vi "Execute.vi"(8 "error in (no error)":errorcluster, 10 "Shifted Error in":refnum<class "Error.lvclass">, 11 "ERROR_Prompt in":refnum<class "ERROR_Prompt.lvclass">) -> (0 "error out":errorcluster, 1 "STOP?":bool, 2 "Shifted Error out":refnum<class "Error.lvclass">, 3 "ERROR_Prompt out":refnum<class "ERROR_Prompt.lvclass">)   [LabVIEW 2019, in "TSC Error.lvlib" / "ERROR_Prompt.lvclass"]
doc: "The Error Prompt function will send a message using the queue reference to the application for the error that happened in the software.\n\nInputs:\n-ERROR_Prompt in [obj] - the dynamic dispatch input class\n-Shifted Error in [obj] - the shifted error class with shared information\n-error in\n\nOutputs:\n-ERROR_Prompt out [obj] - the dynamic dispatch output class\n-Shifted Error in [obj] - the shifted error class with shared information\n-STOP? [Boolean] - the output Boolean used to stop the Error Loop\n-error out\n\n<b>Code Developed By:</b>\nDaniel Coons\nTechnology Service Corporation\n1983 S Liberty Drive\nBloomington, IN 47403\nPhone: 812 558-7100\nwww.tsc.com\\atcs"
uses:
  ERROR_Prompt.lvclass
  C:/Development/Open Source/tsc-error-library/_Messages/Error/Error.lvclass
  Error/Error.lvclass
  <vilib>/Utility/error.llb/DialogType.ctl
  Error/Error.lvclass/Error.ctl
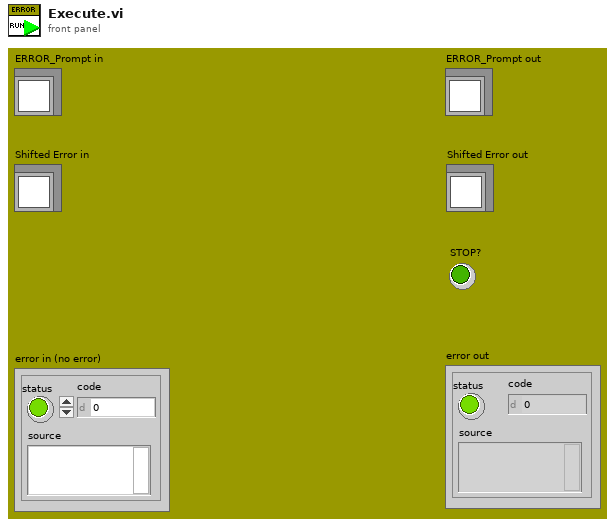
[diagram p1: front panel]
types:
  T1 = typedef "DialogType.ctl" = u16
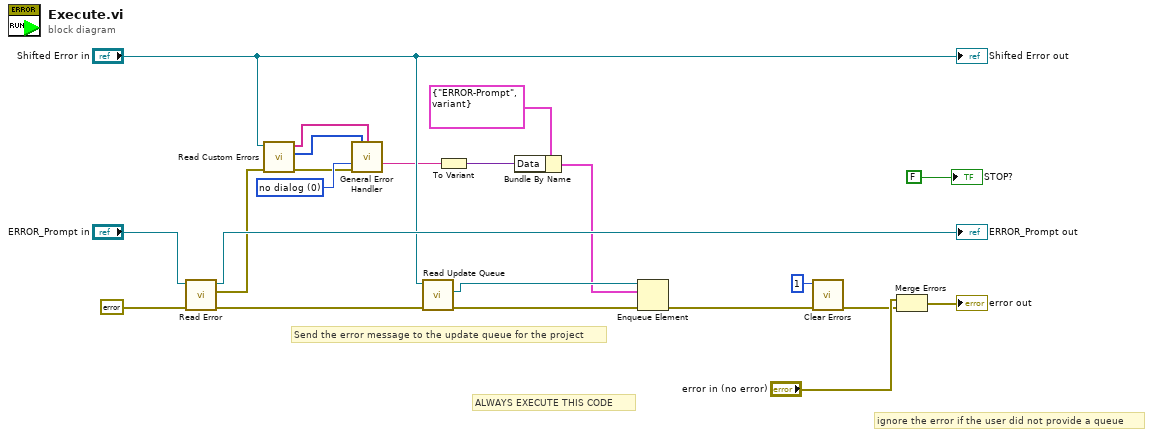
[diagram p0: block diagram]
diagram:
  w20 = T1 0 items=["no dialog", "OK message", "continue or stop message", "OK message + warnings", "continue/stop + warnings"] ("type of dialog (OK msg:1)")
  # "ignore the error if the user did not provide a queue"
  # "Send the error message to the update queue for the project"
  # "ALWAYS EXECUTE THIS CODE"
  n1 = call "Read Error.vi"("error in"=errorcluster {"status"=FALSE, "code"=0, "source"=""} ("error in (no error)"), "Error in"="ERROR_Prompt in") -> ("error out"=w9:errorcluster, "Error"=w19:errorcluster, "Error out"=→"ERROR_Prompt out":refnum<class "ERROR_Prompt.lvclass">)  [unwired: 7 in]
  n2 = call "Read Custom Errors.vi"("Error In"=w19, "Error.lvclass"="Shifted Error in") -> ("Error Out"=w18:errorcluster, "Error Codes"=w16:i32[], "Error Messages"=w17:string[])  [unwired: 7 in]
  n3 = call <vilib>:"General Error Handler.vi"("[user-defined codes]"=w16, "[user-defined descriptions]"=w17, "type of dialog (OK msg:1)"=w20, "error in (no error)"=w18) -> ("message"=w5:string)  [unwired: 7 in, 4 out]
  n4 = call "Read Update Queue.vi"("error in (no error)"=w9, "Error in"="Shifted Error in") -> ("error out"=w10:errorcluster, "Update Queue"=w7:refnum<queue>)  [unwired: 7 in, 1 out]
  n5 = To Variant(anything=w5) -> (Variant=w4:variant)
  n6 = Bundle By Name(cluster=cluster{"Message":string, "Data":variant} {"Message"="ERROR-Prompt", "Data"=variant} ("element"), "Data"=w4) -> (w3:cluster{"Message":string, "Data":variant})
  n7 = Enqueue Element(queue=w7, element=w3, error in (no error)=w10) -> (error out=w8:errorcluster)  [unwired: 1 in, 2 out]
  n8 = call <vilib>:"Clear Errors.vi"("error in (no error)"=w8, "specific error code to clear (0: all)"=1 ("Error Code")) -> ("error out"=w2:errorcluster)  [unwired: 4 in, 1 out]
  n9 = Merge Errors("error in (no error)", w2) -> (→"error out":errorcluster)
  "STOP?" <- FALSE ("STOP?")
  "Shifted Error out" <- "Shifted Error in"
